vi "XBMC Method String Array Params.vi"(7 "id":i32=1, 8 "Error In":errorcluster, 9 "params":cluster{"action":string}, 10 "method":string, 11 "jsonrpc":string="2.0") -> (0 "Error Out":errorcluster, 3 "JSON Request":string)   [LabVIEW 2013, in "LMH-Kodi.lvlib"]
uses:
  LMH-Kodi.lvlib
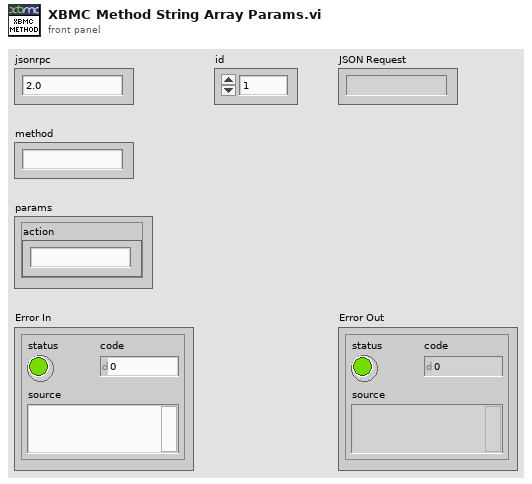
[diagram p1: front panel]
types:
  T1 = cluster{"jsonrpc":string, "method":string, "params":cluster{"action":string}, "id":i32}
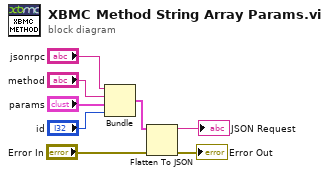
[diagram p0: block diagram]
diagram:
  n1 = Bundle("jsonrpc"="jsonrpc", "method"="method", "params"="params", "id"="id") -> (w7:T1)  [unwired: 1 in]
  n2 = Flatten To JSON(anything=w7, error in (no error)="Error In") -> (JSON string=→"JSON Request":string, 11:→"Error Out":errorcluster)  [unwired: 1 in]
